vi "Read ids.vi"(8 "error in (no error)":errorcluster, 11 "JSON-RPC in":refnum<class "JSON-RPC.lvclass">) -> (0 "error out":errorcluster, 2 "ids":string[](array[string]), 3 "JSON-RPC out":refnum<class "JSON-RPC.lvclass">)   [LabVIEW 2019, in "JSON-RPC.lvclass"]
uses:
  JSON-RPC.lvclass
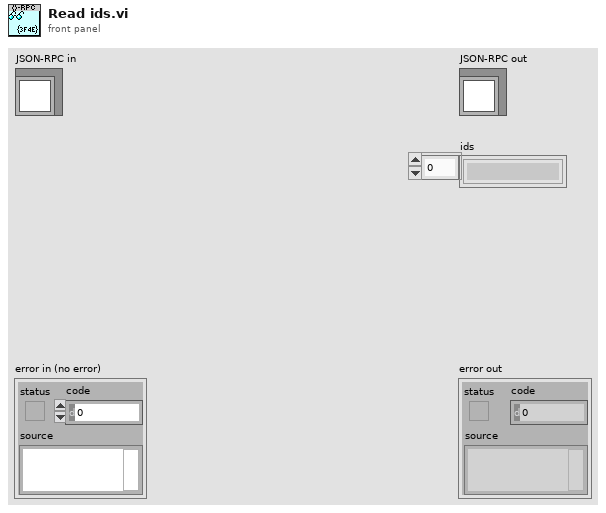
[diagram p1: front panel]
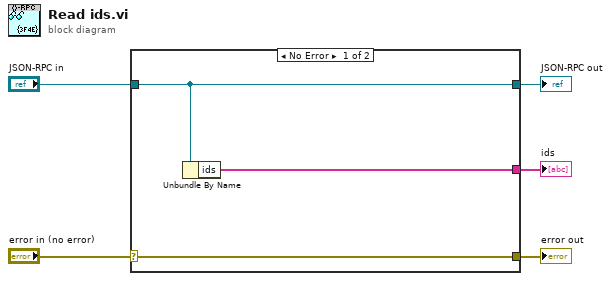
[diagram p0: block diagram]
diagram:
  n1 = case shown="No Error" "error in (no error)" {
    selector: "error in (no error)" -> [w8 w9]
    tunnel: [w8 w9] -> w4
    tunnel: [w6 w10] -> w2
    tunnel: "JSON-RPC in" -> [w6 w10]
    tunnel: [w7 _] -> w1
    frame No Error {
      n2 = Unbundle By Name(w6) -> ("ids"=w7:string[])
    }
    frame Error {
    }
  }
  "error out" <- w4
  "JSON-RPC out" <- w2
  "ids" <- w1
